vi "SimpleBenchmark.vi"() -> ()   [LabVIEW 2023]
uses:
  <vilib>/Analysis/NI_AALBase.lvlib
  x64/Release/libMed.dll
panel:
  out "Nth Res":dbl[](array[numeric])
  out "Passed 2":bool[](array[boolean])=[TRUE, TRUE, TRUE]
  out "Nth Median, ms":dbl[](array[numeric])=[6.021880000000124, 23.395960000001992, 92.48405000000162]
  in  "NaN Test":bool
  out "My Res":dbl[](array[numeric])
  out "NI Median Res":dbl[](array[numeric])
  out "My Median, ms":dbl[](array[numeric])=[6.021880000000124, 23.395960000001992, 92.48405000000162]
  out "NI Median, ms":dbl[](array[numeric])=[15.592999999995527, 49.55369999998993, 197.07800000000475]
  out "Passed":bool[](array[boolean])=[TRUE, TRUE, TRUE]
  # ">python fastMedTest.py\nMy 1M: 5.95 ms c_double(0.5002955)\nnp 1M: 10.97 ms 0.5002955\npassed\nMy 4M: 18.45 ms c_double(0.49972385)\nnp 4M: 47.87 ms 0.49972385\npassed\nMy 16M: 80.29 ms c_double(0.50009161)\nnp 16M: 181.33 ms 0.50009161\npassed"
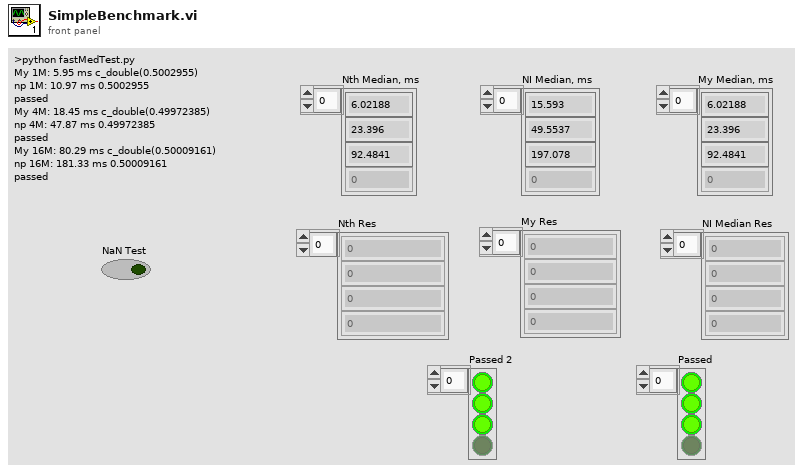
[diagram p1: front panel]
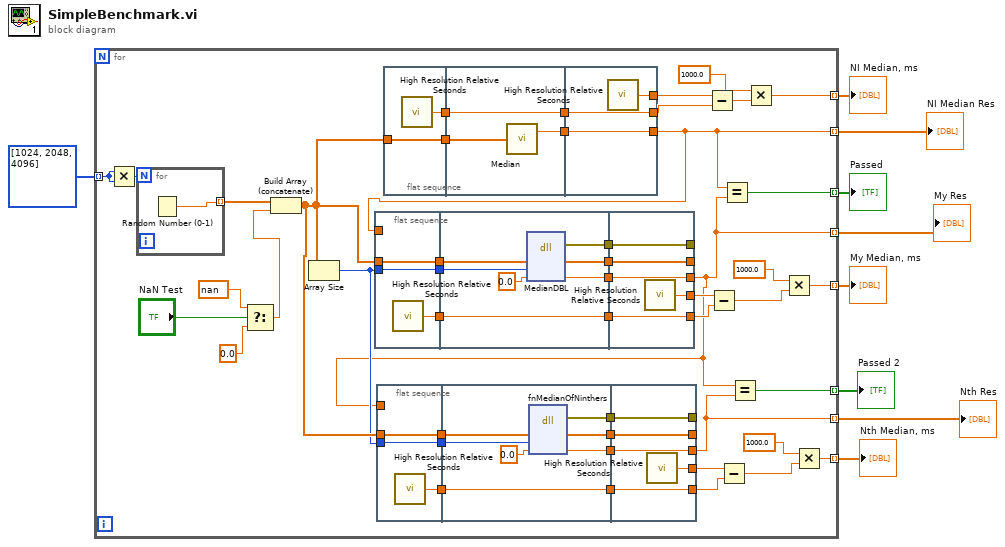
[diagram p0: block diagram]
diagram:
  n1 = for {
    tunnel: i32[] [1024, 2048, 4096] -> [w50] mode=indexing
    tunnel: [w49] -> w8 mode=indexing
    tunnel: [w47] -> w7 mode=indexing
    tunnel: [w37] -> w6 mode=indexing
    tunnel: [w13] -> w5 mode=indexing
    tunnel: [w14] -> w4 mode=indexing
    tunnel: [w19] -> w3 mode=indexing
    tunnel: [w15] -> w2 mode=indexing
    tunnel: [w12] -> w1 mode=indexing
    n2 = Multiply(x=w50, y=w50) -> (x*y=w21:i32)
    n3 = for {
      N: w21 -> [_]
      tunnel: [w95] -> w10 mode=indexing
      n4 = Random Number (0-1)() -> (number: 0 to 1=w95:dbl)
    }
    n5 = Select(t=nan, s="NaN Test", f=0.0) -> (s? t:f=w11:dbl)
    n6 = Build Array (concatenate)(w10, w11) -> (w23:dbl[])
    n7 = Array Size(array=w23) -> (size(s)=w22:i32)
    n8 = flat-sequence {
      tunnel: w23 -> [w74]
      tunnel: [w74] -> w53
      tunnel: [w73] -> w40
      tunnel: w22 -> [w72]
      tunnel: [w72] -> w39
      tunnel: w13 -> [_]
      tunnel: w53 -> [w81]
      tunnel: [w80] -> w52
      tunnel: [w79] -> w41
      tunnel: w40 -> [w79]
      tunnel: w39 -> [w78]
      tunnel: [w77] -> w35
      tunnel: [w76] -> w34
      tunnel: [w86] -> w14
      tunnel: w52 -> [w86]
      tunnel: [w85] -> w51
      tunnel: [w84] -> w42
      tunnel: w41 -> [w84]
      tunnel: [w83] -> _
      tunnel: w35 -> [w83]
      tunnel: [w82] -> _
      tunnel: w34 -> [w82]
      frame #0 {
        n9 = call <vilib>:"High Resolution Relative Seconds.vi"() -> ("relative seconds"=w73:dbl)
      }
      frame #1 {
        n10 = dll-call lib="C:/Users/Andrey/Desktop/fastMed/src/x64/Release/libMed.dll" fn="MedianDBL"("xH"=w81, "size"=w78, "median"=0.0) -> (error out=w77:errorcluster, "xH"=w76:dbl[], "median"=w80:dbl)  [unwired: 5 in, 1 out]
      }
      frame #2 {
        n11 = call <vilib>:"High Resolution Relative Seconds.vi"() -> ("relative seconds"=w85:dbl)
      }
    }
    n12 = flat-sequence {
      tunnel: w23 -> [w59]
      tunnel: [w59] -> w30
      tunnel: [w58] -> w29
      tunnel: w22 -> [w57]
      tunnel: [w57] -> w28
      tunnel: w14 -> [_]
      tunnel: w30 -> [w66]
      tunnel: [w65] -> w27
      tunnel: [w64] -> w26
      tunnel: w29 -> [w64]
      tunnel: w28 -> [w63]
      tunnel: [w62] -> w25
      tunnel: [w61] -> w24
      tunnel: [w71] -> w12
      tunnel: w27 -> [w71]
      tunnel: [w70] -> w17
      tunnel: [w69] -> w16
      tunnel: w26 -> [w69]
      tunnel: [w68] -> _
      tunnel: w25 -> [w68]
      tunnel: [w67] -> _
      tunnel: w24 -> [w67]
      frame #0 {
        n13 = call <vilib>:"High Resolution Relative Seconds.vi"() -> ("relative seconds"=w58:dbl)
      }
      frame #1 {
        n14 = dll-call lib="C:/Users/Andrey/Desktop/fastMed/src/x64/Release/libMed.dll" fn="fnMedianOfNinthers"("xH"=w66, "size"=w63, "median"=0.0) -> (error out=w62:errorcluster, "xH"=w61:dbl[], "median"=w65:dbl)  [unwired: 5 in, 1 out]
      }
      frame #2 {
        n15 = call <vilib>:"High Resolution Relative Seconds.vi"() -> ("relative seconds"=w70:dbl)
      }
    }
    n16 = flat-sequence {
      tunnel: w23 -> [w88]
      tunnel: [w88] -> w56
      tunnel: [w87] -> w43
      tunnel: w56 -> [w91]
      tunnel: [w90] -> w55
      tunnel: [w89] -> w44
      tunnel: w43 -> [w89]
      tunnel: [w94] -> w13
      tunnel: w55 -> [w94]
      tunnel: [w93] -> w54
      tunnel: [w92] -> w45
      tunnel: w44 -> [w92]
      frame #0 {
        n17 = call <vilib>:"High Resolution Relative Seconds.vi"() -> ("relative seconds"=w87:dbl)
      }
      frame #1 {
        n18 = call <vilib>:"Median.vi"("X"=w91) -> ("median"=w90:dbl)  [unwired: 1 out]
      }
      frame #2 {
        n19 = call <vilib>:"High Resolution Relative Seconds.vi"() -> ("relative seconds"=w93:dbl)
      }
    }
    n20 = Subtract(x=w54, y=w45) -> (x-y=w48:dbl)
    n21 = Subtract(x=w51, y=w42) -> (x-y=w38:dbl)
    n22 = Subtract(x=w17, y=w16) -> (x-y=w18:dbl)
    n23 = Equal?(x=w13, y=w14) -> (x = y?=w49:bool)
    n24 = Equal?(x=w14, y=w12) -> (x = y?=w15:bool)
    n25 = Multiply(x=1000.0, y=w48) -> (x*y=w47:dbl)
    n26 = Multiply(x=1000.0, y=w38) -> (x*y=w37:dbl)
    n27 = Multiply(x=1000.0, y=w18) -> (x*y=w19:dbl)
  }
  "Passed" <- w8
  "NI Median, ms" <- w7
  "My Median, ms" <- w6
  "NI Median Res" <- w5
  "My Res" <- w4
  "Nth Median, ms" <- w3
  "Passed 2" <- w2
  "Nth Res" <- w1
